vi "Set Shared Class.vi"(0 "gen in":refnum<class "niUSRP Tx DSP v2 FPGA.lvclass">=refnum, 5 "shared":refnum<class "niVST Shared v1 FPGA.lvclass">=refnum) -> (4 "gen out":refnum<class "niUSRP Tx DSP v2 FPGA.lvclass">)   [LabVIEW 2023]
uses:
  <instrlib>/niVST/Reference FPGA/FPGA/Shared/v1/niVST Shared v1 FPGA.lvclass
  <instrlib>/niUSRP/Reference FPGA/Tx DSP/niUSRP Tx DSP v2 FPGA.lvclass
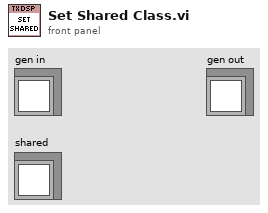
[diagram p1: front panel]
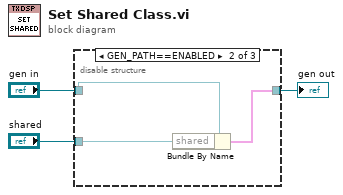
[diagram p0: block diagram]
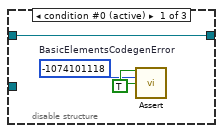
[diagram p2: hidden frame]
diagram:
  n1 = disable-structure shown="GEN_PATH==ENABLED" {
    disable-tunnel: "gen in" -> [w4 w9 w10]
    disable-tunnel: [w4 w8 w10] -> w2
    disable-tunnel: "shared" -> [_ w7 _]
    frame condition #0 (active) {
      w6 = TRUE ("assert")
      w5 = -1074101118  # BasicElementsCodegenError
      n2 = call <instrlib>:"Assert.vi"("assert"=w6, "error code"=w5, "enable show error"=w6) -> ()  [unwired: 13 in]
    }
    frame condition #1 {
      n3 = Bundle By Name(cluster=w9, "shared"=w7) -> (w8:cluster{})
    }
    frame condition #2 {
    }
  }
  "gen out" <- w2
